vi "Process Data.vi"(8 "error in (no error)":errorcluster, 10 "Data In":string, 11 "Data Cluster in":T1={"Data Display"="", "FP Control Refs"={"Connect to Station Ref"=refnum, "Download Ref"=refnum, "Exit Button Ref"=refnum, "Start Date Refnum"=refnum, "End Date Refnum"=refnum, "Path"=refnum, "COM Port"="", "IP or Phone Ref"=refnum, "TCPIP ID"=refnum, "Reboot Refnum"=refnum, "Datafile Refnum"=refnum}, "FP Indicator Refs"={"Connected Refnum"=refnum, "Data Display Ref"=refnum, "Station ID Ref"=refnum}, "User Events"={"Stop"=refnum, "Update Display"=refnum}, "Message Queues"={"UI"=refnum, "ACQUISITION"=refnum, "PROCESSING"=refnum, "LOGGING"=refnum}, "IS IP?"=FALSE, "Downloading?"=FALSE, "DCP Version"=enum."XPert2", "Processing Loop State"=enum."Get Station  ID", "Username"=refnum, "Password"=refnum}) -> (0 "error out":errorcluster, 3 "Data Cluster out":T1={"Data Display"="", "FP Control Refs"={"Connect to Station Ref"=refnum, "Download Ref"=refnum, "Exit Button Ref"=refnum, "Start Date Refnum"=refnum, "End Date Refnum"=refnum, "Path"=refnum, "COM Port"="", "IP or Phone Ref"=refnum, "TCPIP ID"=refnum, "Reboot Refnum"=refnum, "Datafile Refnum"=refnum}, "FP Indicator Refs"={"Connected Refnum"=refnum, "Data Display Ref"=refnum, "Station ID Ref"=refnum}, "User Events"={"Stop"=refnum, "Update Display"=refnum}, "Message Queues"={"UI"=refnum, "ACQUISITION"=refnum, "PROCESSING"=refnum, "LOGGING"=refnum}, "IS IP?"=FALSE, "Downloading?"=FALSE, "DCP Version"=enum."XPert2", "Processing Loop State"=enum."Get Station  ID", "Username"=refnum, "Password"=refnum})   [LabVIEW 2018]
uses:
  controls/GLDL UI Data.ctl
  controls/Disconnect Control.ctl
  controls/Download Control.ctl
  controls/Exit Control.ctl
  controls/Date Control.ctl
  controls/IP Phone Number Control.ctl
  controls/Reboot Control.ctl
  controls/Connected Indicator.ctl
  controls/Output Indicator.ctl
  controls/Station ID Indicator.ctl
  Message Queue/All Message Queues.ctl
  Message Queue/Message Cluster.ctl
  controls/Processing Loop State.ctl
  Message Queue/Enqueue Message (Single).vi
  Message Queue/GLDL Message Queue.lvlib
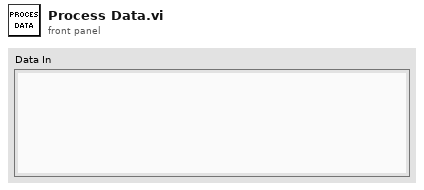
[diagram p1: front panel]
types:
  T1 = typedef "GLDL UI Data.ctl" = cluster{"Data Display":string, "FP Control Refs":cluster{"Connect to Station Ref":refnum<vi>, "Download Ref":refnum<vi>, "Exit Button Ref":refnum<vi>, "Start Date Refnum":refnum<vi>, "End Date Refnum":refnum<vi>, "Path":refnum<vi>, "COM Port":refnum<visa-resource-name>, "IP or Phone Ref":refnum<vi>, "TCPIP ID":refnum<k5>, "Reboot Refnum":refnum<vi>, "Datafile Refnum":refnum<file>}, "FP Indicator Refs":cluster{"Connected Refnum":refnum<vi>, "Data Display Ref":refnum<vi>, "Station ID Ref":refnum<vi>}, "User Events":cluster{"Stop":refnum<user-event>, "Update Display":refnum<user-event>}, "Message Queues":T2, "IS IP?":bool, "Downloading?":bool, "DCP Version":enum16{"XPert", "XPert2"}, "Processing Loop State":T3, "Username":refnum<vi>, "Password":refnum<vi>}
  T2 = typedef "GLDL Message Queue.lvlib/All Message Queues.ctl" = cluster{"UI":refnum<queue>, "ACQUISITION":refnum<queue>, "PROCESSING":refnum<queue>, "LOGGING":refnum<queue>}
  T3 = typedef "Processing Loop State.ctl" = enum16{"Get Station  ID", "Change Directory SD Card", "Change Directory Storage Card", "Downloading", "Idle in DL Directory"}
  T4 = typedef "Connected Indicator.ctl" = bool
  T5 = enum16{"open", "replace", "create", "open or create", "replace or create", "replace or create with confirmation"}
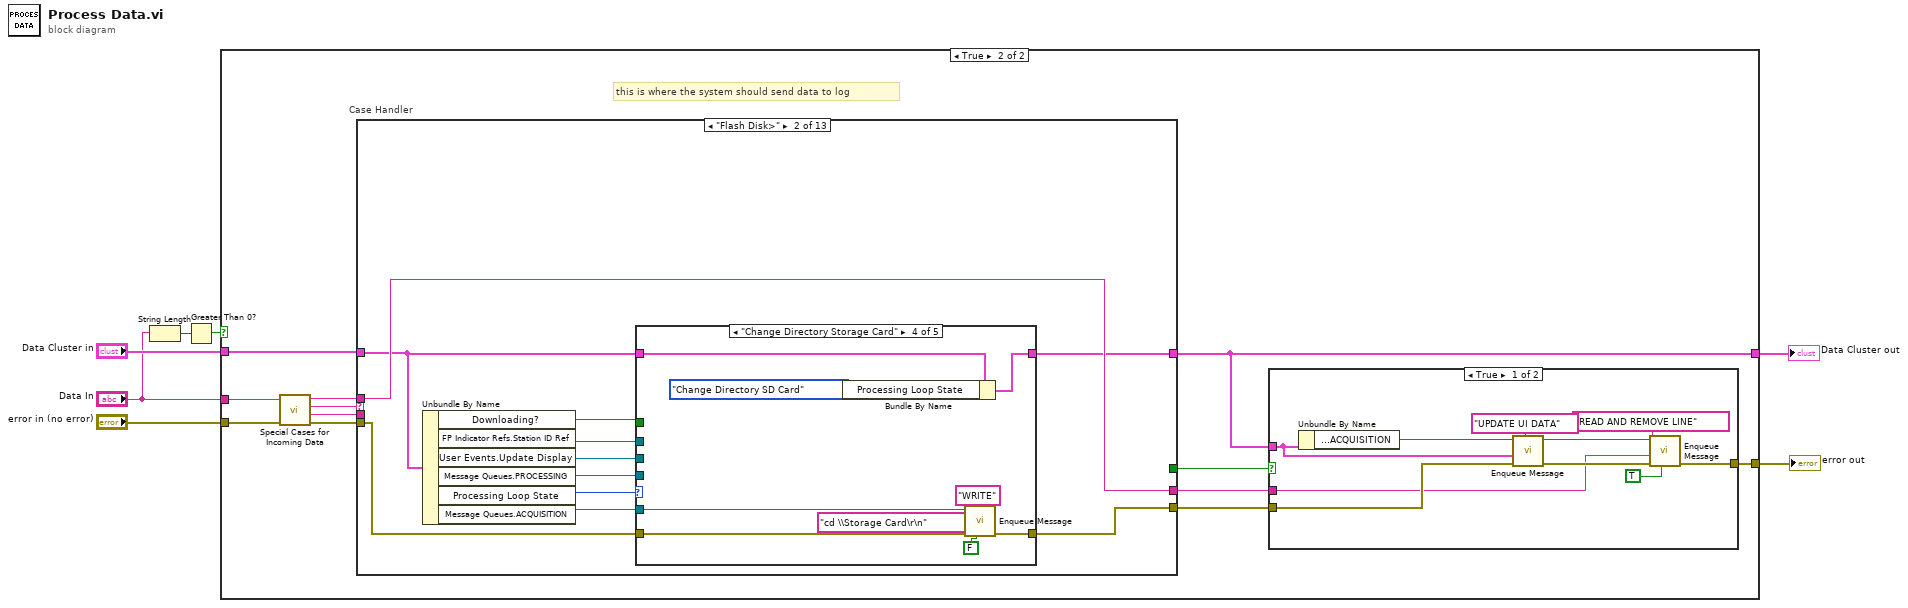
[diagram p0: block diagram]
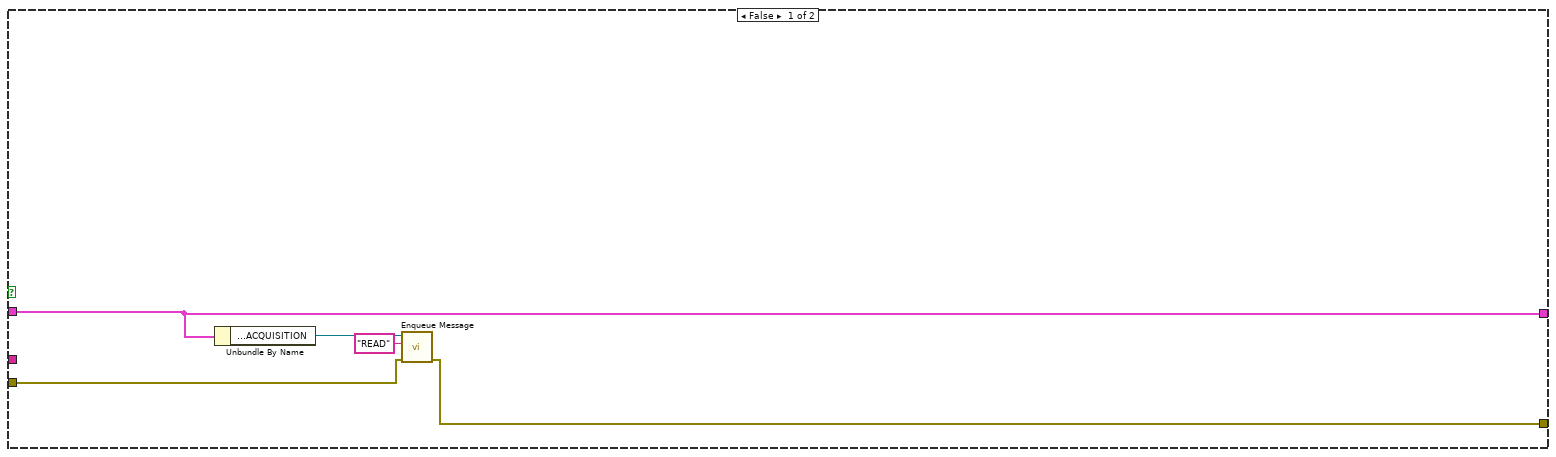
[diagram p2: hidden frame]
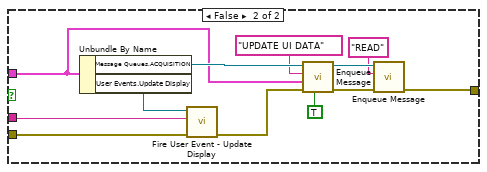
[diagram p3: hidden frame]
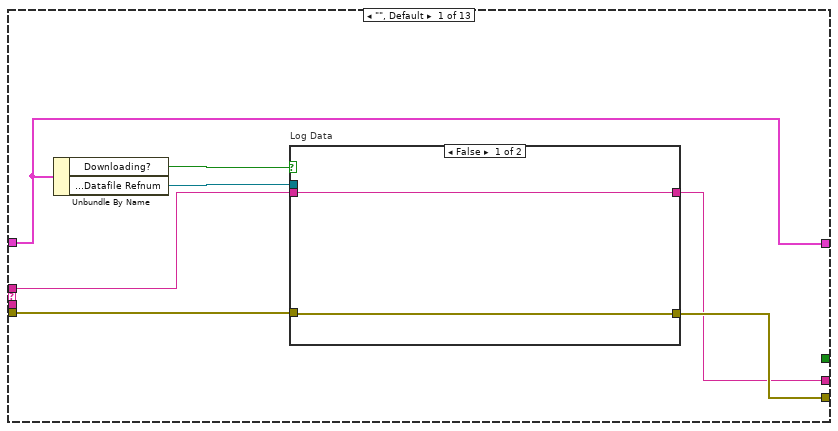
[diagram p4: hidden frame]
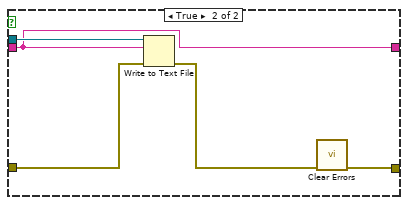
[diagram p5: hidden frame]
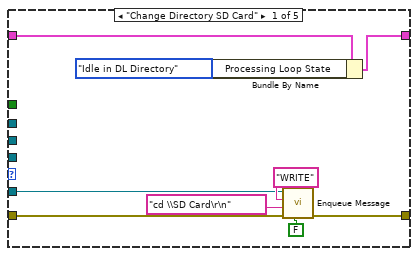
[diagram p6: hidden frame]
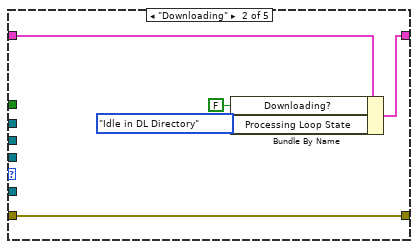
[diagram p7: hidden frame]
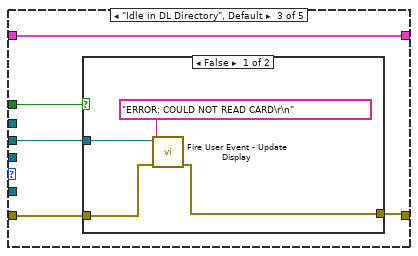
[diagram p8: hidden frame]
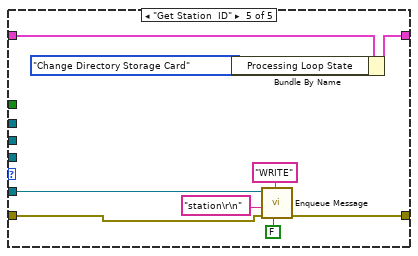
[diagram p10: hidden frame]
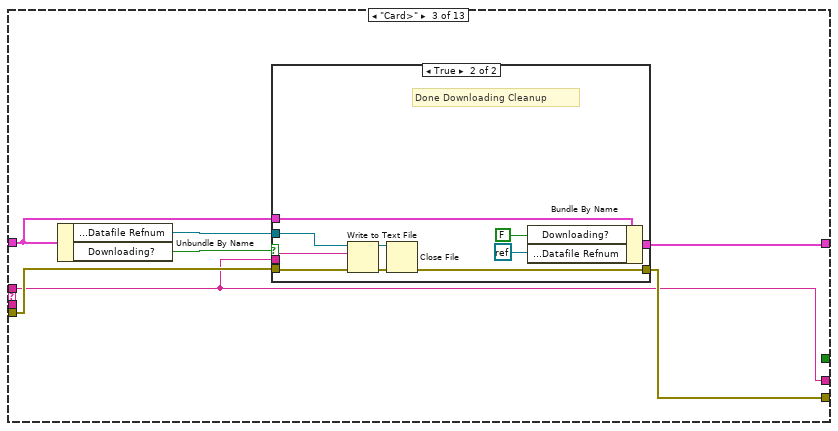
[diagram p11: hidden frame]
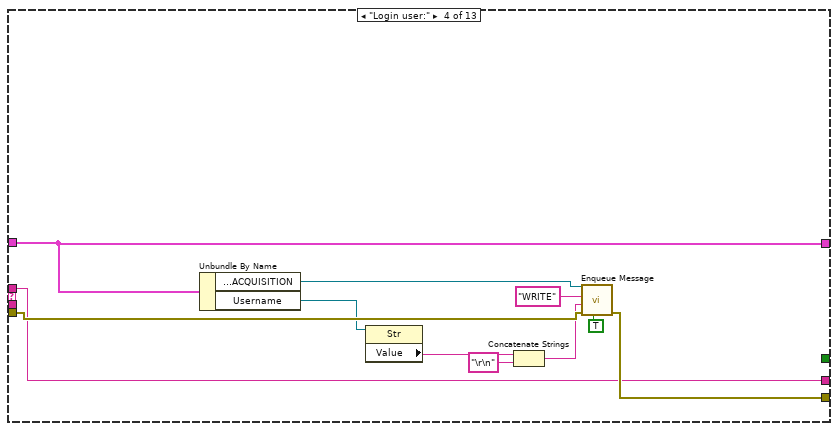
[diagram p13: hidden frame]
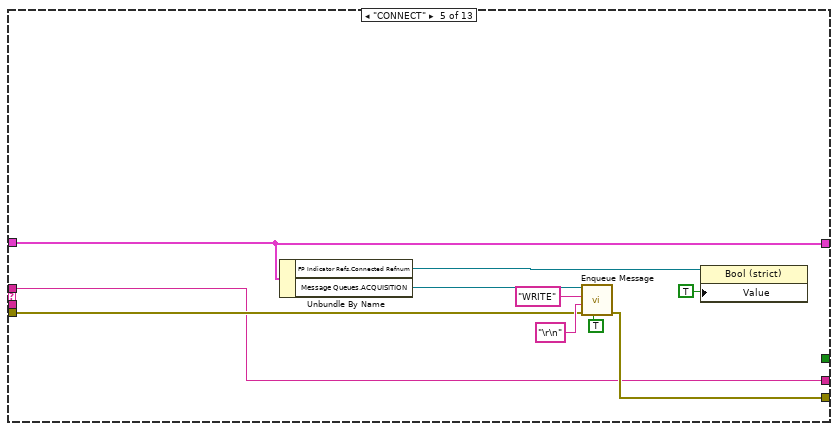
[diagram p14: hidden frame]
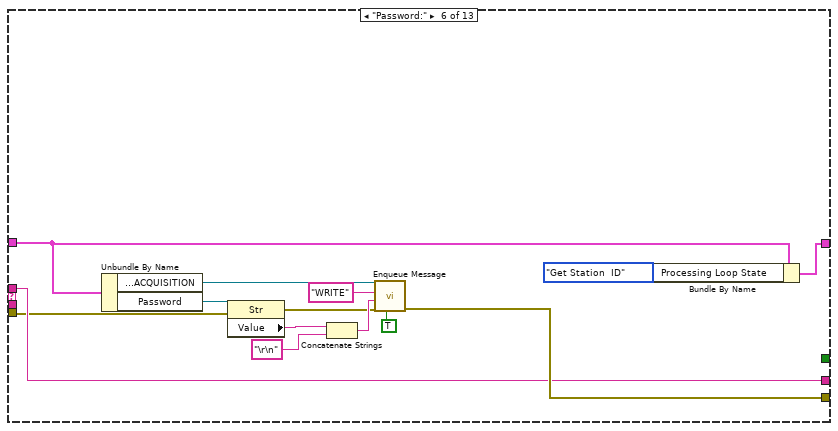
[diagram p15: hidden frame]
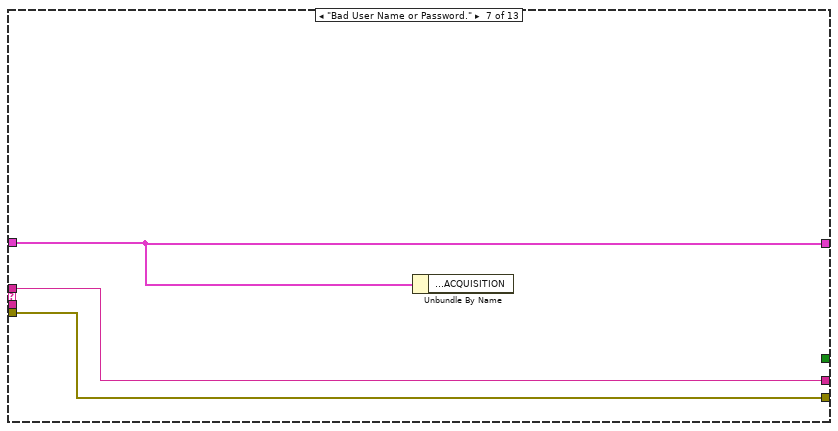
[diagram p16: hidden frame]
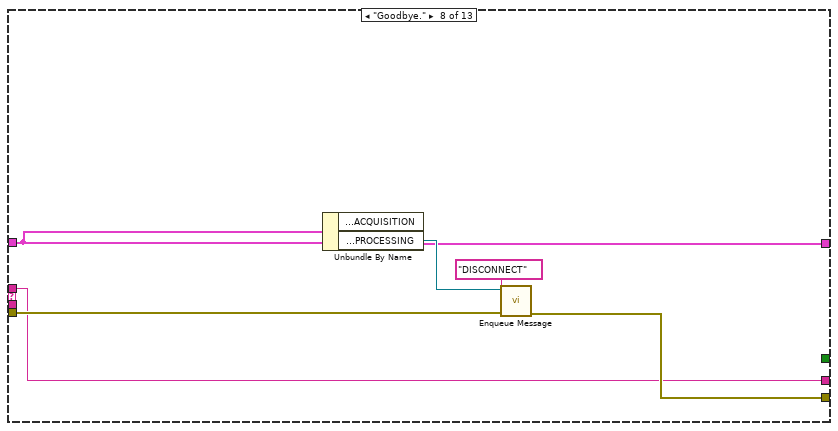
[diagram p17: hidden frame]
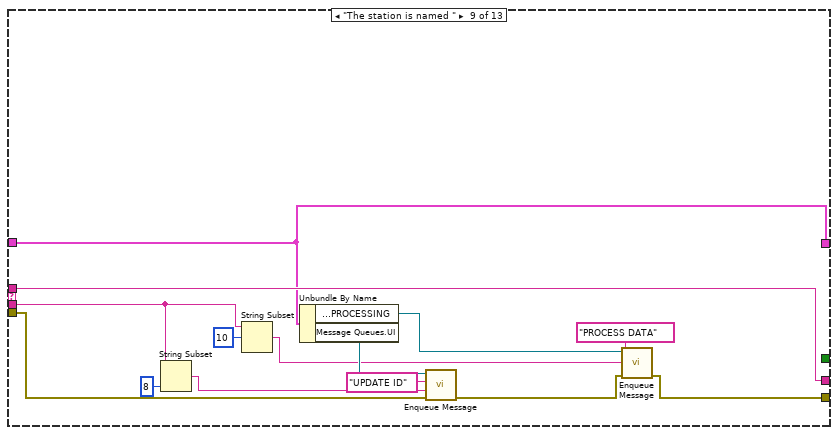
[diagram p18: hidden frame]
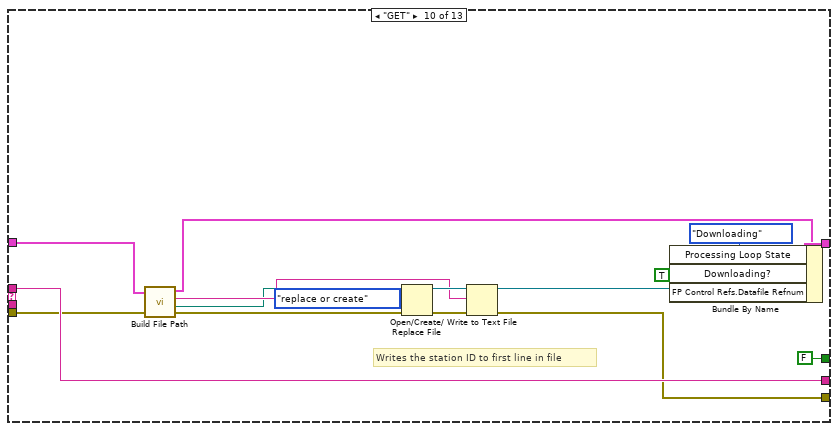
[diagram p19: hidden frame]
diagram:
  n1 = String Length(string="Data In") -> (length=w3:i32)
  n2 = Greater Than 0?(x=w3) -> (x > 0?=w2:bool)
  n3 = case shown="True" w2 {
    tunnel: "error in (no error)" -> [w9 w20]
    tunnel: [w8 w24] -> w5
    tunnel: "Data In" -> [_ w23]
    tunnel: "Data Cluster in" -> [w12 w18]
    tunnel: [w12 w13] -> w7
    frame False {
      n4 = Unbundle By Name(w12) -> ("Message Queues.ACQUISITION"=w11:refnum<queue>)
      n5 = call-poly "Enqueue Message.vi"("error in (no error)"=w9, "Message"="READ", "Message Queue"=w11) -> ("error out"=w8:errorcluster)  [unwired: 7 in, 1 out]
    }
    frame True {
      # "this is where the system should send data to log"
      n6 = call "Special Cases for Incoming Data.vi"("error in (no error)"=w20, "Data In"=w23) -> ("error out"=w22:errorcluster, "After Special Case"=w16:string, "Special Case"=w15:string, "Data Out"=w21:string)  [unwired: 5 in, 1 out]
      n7 = case "Case Handler" shown="\"Flash Disk>\"" w15 {
        tunnel: w22 -> [w50 w71 w116 w140 w149 w154 w170 w176 w185 w201 w207 w214 w225]
        tunnel: [w49 w63 w115 w141 w150 w165 w170 w174 w177 w193 w207 w213 w223] -> w17
        tunnel: w21 -> [w48 w69 w114 w137 w146 w163 w168 w171 w190 w206 w209 w219 w228]
        tunnel: w18 -> [w53 w66 w119 w139 w148 w162 w169 w172 w184 w203 w208 w218 w227]
        tunnel: [w47 w69 w114 w137 w146 w163 w168 w171 w190 w206 w209 w217 w228] -> w19
        tunnel: [w53 w65 w118 w139 w148 w161 w169 w172 w184 w204 w208 w218 w227] -> w13
        tunnel: w16 -> [_ _ _ _ _ _ _ _ w181 _ _ _ _]
        tunnel: [_ _ _ _ _ _ _ _ _ FALSE _ TRUE _] -> w14
        frame "", Default {
          n8 = Unbundle By Name(w53) -> ("Downloading?"=w52:bool, "FP Control Refs.Datafile Refnum"=w51:refnum<file>)
          n9 = case "Log Data" shown="False" w52 {
            tunnel: w51 -> [_ w60]
            tunnel: w50 -> [w55 w59]
            tunnel: [w55 w56] -> w49
            tunnel: w48 -> [w54 w58]
            tunnel: [w54 w58] -> w47
            frame False {
            }
            frame True {
              n10 = Write to Text File(file (use dialog)=w60, text=w58, error in=w59) -> (error out=w57:errorcluster)  [unwired: 1 in, 2 out]
              n11 = call <vilib>:"Clear Errors.vi"("error in (no error)"=w57) -> ("error out"=w56:errorcluster)  [unwired: 5 in, 1 out]
            }
          }
        }
        frame "Flash Disk>" {
          # "Get Station Number"
          n12 = Unbundle By Name(w66) -> ("Downloading?"=w61:bool, "FP Indicator Refs.Station ID Ref"=w62:refnum<vi>, "User Events.Update Display"=w64:refnum<user-event>, "Message Queues.PROCESSING"=w67:refnum<queue>, "Processing Loop State"=w68:T3, "Message Queues.ACQUISITION"=w70:refnum<queue>)
          n13 = case shown="\"Change Directory Storage Card\"" w68 {
            tunnel: w71 -> [w72 w85 w88 w96 w105]
            tunnel: w70 -> [w73 _ _ w97 w106]
            tunnel: [w74 w85 w87 w98 w107] -> w63
            tunnel: w67 -> [_ _ _ _ _]
            tunnel: w66 -> [w80 w84 w90 w104 w112]
            tunnel: [w79 w83 w90 w103 w113] -> w65
            tunnel: w64 -> [_ _ w89 _ _]
            tunnel: w62 -> [_ _ _ _ _]
            tunnel: w61 -> [_ _ w86 _ _]
            frame "Change Directory SD Card" {
              n14 = Bundle By Name(cluster=w80, "Processing Loop State"=Processing_Loop_State."Idle in DL Directory") -> (w79:T1)
              n15 = call-poly "Enqueue Message.vi"("Priority Message? (F)"=FALSE, "error in (no error)"=w72, "Message Data"="cd \\SD Card\r\n" ("Initial Message"), "Message"="WRITE" ("Initial Message"), "Message Queue"=w73) -> ("error out"=w74:errorcluster)  [unwired: 5 in, 1 out]
            }
            frame "Downloading" {
              n16 = Bundle By Name(cluster=w84, "Downloading?"=FALSE, "Processing Loop State"=Processing_Loop_State."Idle in DL Directory") -> (w83:T1)
            }
            frame "Idle in DL Directory", Default {
              n17 = case shown="False" w86 {
                tunnel: w89 -> [w94 _]
                tunnel: w88 -> [w93 w95]
                tunnel: [w91 w95] -> w87
                frame False {
                  n18 = call "Fire User Event - Update Display.vi"("error in (no error)"=w93, "event data"="ERROR: COULD NOT READ CARD\r\n" ("Initial Message"), "Update Display"=w94) -> ("error out"=w91:errorcluster)  [unwired: 8 in]
                }
                frame True {
                }
              }
            }
            frame "Change Directory Storage Card" {
              n19 = Bundle By Name(cluster=w104, "Processing Loop State"=Processing_Loop_State."Change Directory SD Card") -> (w103:T1)
              n20 = call-poly "Enqueue Message.vi"("Priority Message? (F)"=FALSE, "error in (no error)"=w96, "Message Data"="cd \\Storage Card\r\n" ("data in"), "Message"="WRITE" ("Initial Message"), "Message Queue"=w97) -> ("error out"=w98:errorcluster)  [unwired: 5 in, 1 out]
            }
            frame "Get Station  ID" {
              n21 = Bundle By Name(cluster=w112, "Processing Loop State"=Processing_Loop_State."Change Directory Storage Card") -> (w113:T1)
              n22 = call-poly "Enqueue Message.vi"("Priority Message? (F)"=FALSE, "error in (no error)"=w105, "Message Data"="station\r\n" ("data in"), "Message"="WRITE" ("Initial Message"), "Message Queue"=w106) -> ("error out"=w107:errorcluster)  [unwired: 5 in, 1 out]
            }
          }
        }
        frame "Card>" {
          n23 = Unbundle By Name(w119) -> ("FP Control Refs.Datafile Refnum"=w117:refnum<file>, "Downloading?"=w120:bool)
          n24 = case shown="True" w120 {
            tunnel: w119 -> [w122 w132]
            tunnel: [w122 w130] -> w118
            tunnel: w117 -> [_ w128]
            tunnel: w116 -> [w121 w125]
            tunnel: [w121 w124] -> w115
            tunnel: w114 -> [_ w123]
            frame False {
              # "Not Done Downloading"
            }
            frame True {
              # "Done Downloading Cleanup"
              n25 = Write to Text File(file (use dialog)=w128, text=w123, error in=w125) -> (refnum out=w127:refnum<file>, error out=w126:errorcluster)  [unwired: 1 in, 1 out]
              n26 = Close File(refnum=w127, error in=w126) -> (error out=w124:errorcluster)  [unwired: 1 out]
              n27 = Bundle By Name(cluster=w132, "Downloading?"=FALSE, "FP Control Refs.Datafile Refnum"=refnum<k0> refnum) -> (w130:T1)
            }
          }
        }
        frame "Login user:" {
          n28 = Unbundle By Name(w139) -> ("Message Queues.ACQUISITION"=w138:refnum<queue>, "Username"=w136:refnum<vi>)
          n29 = property class="Str"(reference=w136) -> ("Value"=w135:string)  [unwired: 1 in, 2 out]
          n30 = Concatenate Strings(w135, "\r\n" ("write buffer")) -> (w133:string)
          n31 = call-poly "Enqueue Message.vi"("Priority Message? (F)"=TRUE, "error in (no error)"=w140, "Message Data"=w133, "Message"="WRITE" ("Initial Message"), "Message Queue"=w138) -> ("error out"=w141:errorcluster)  [unwired: 5 in, 1 out]
        }
        frame "CONNECT" {
          n32 = Unbundle By Name(w148) -> ("FP Indicator Refs.Connected Refnum"=w145:refnum<vi>, "Message Queues.ACQUISITION"=w147:refnum<queue>)
          n33 = call-poly "Enqueue Message.vi"("Priority Message? (F)"=TRUE, "error in (no error)"=w149, "Message Data"="\r\n" ("write buffer"), "Message"="WRITE" ("Initial Message"), "Message Queue"=w147) -> ("error out"=w150:errorcluster)  [unwired: 5 in, 1 out]
          n34 = property class="Bool (strict)"(reference=w145, "Value"=T4 TRUE) -> ()  [unwired: 1 in, 2 out]
        }
        frame "Password:" {
          # "akl is the only option for now"
          n35 = Unbundle By Name(w162) -> ("Message Queues.ACQUISITION"=w164:refnum<queue>, "Password"=w159:refnum<vi>)
          n36 = property class="Str"(reference=w159, error in=w154) -> (error out=w155:errorcluster, "Value"=w158:string)  [unwired: 1 out]
          n37 = Concatenate Strings(w158, "\r\n" ("write buffer")) -> (w156:string)
          n38 = call-poly "Enqueue Message.vi"("Priority Message? (F)"=TRUE, "error in (no error)"=w155, "Message Data"=w156, "Message"="WRITE" ("Initial Message"), "Message Queue"=w164) -> ("error out"=w165:errorcluster)  [unwired: 5 in, 1 out]
          n39 = Bundle By Name(cluster=w162, "Processing Loop State"=Processing_Loop_State."Get Station  ID") -> (w161:T1)
        }
        frame "Bad User Name or Password." {
          n40 = Unbundle By Name(w169) -> ()  [unwired: 1 out]
        }
        frame "Goodbye." {
          # "Logged out. Now Disconnect"
          n41 = Unbundle By Name(w172) -> ("Message Queues.PROCESSING"=w173:refnum<queue>)  [unwired: 1 out]
          n42 = call-poly "Enqueue Message.vi"("error in (no error)"=w176, "Message"="DISCONNECT", "Message Queue"=w173) -> ("error out"=w174:errorcluster)  [unwired: 7 in, 1 out]
        }
        frame "The station is named " {
          # "Do something with the Station ID"
          n43 = String Subset(string=w181, length (rest)=8 ("length (rest)")) -> (substring=w188:string)  [unwired: 1 in]
          n44 = String Subset(string=w181, offset (0)=10) -> (substring=w179:string)  [unwired: 1 in]
          n45 = Unbundle By Name(w184) -> ("Message Queues.PROCESSING"=w182:refnum<queue>, "Message Queues.UI"=w187:refnum<queue>)
          n46 = call-poly "Enqueue Message.vi"("error in (no error)"=w185, "Message Data"=w188, "Message"="UPDATE ID", "Message Queue"=w187) -> ("error out"=w178:errorcluster)  [unwired: 6 in, 1 out]
          n47 = call-poly "Enqueue Message.vi"("error in (no error)"=w178, "Message Data"=w179, "Message"="PROCESS DATA", "Message Queue"=w182) -> ("error out"=w177:errorcluster)  [unwired: 6 in, 1 out]
        }
        frame "GET" {
          # "Writes the station ID to first line in file"
          n48 = call "Build File Path.vi"("error in (no error)"=w201, "Data Cluster in"=w203) -> ("error out"=w202:errorcluster, "appended path"=w196:path, "Station ID"=w197:string, "Data Cluster out"=w194:T1)  [unwired: 6 in]
          n49 = Open/Create/Replace File(file path (use dialog)=w196, error in=w202, operation (0:open)=T5."replace or create") -> (refnum out=w200:refnum<file>, error out=w199:errorcluster)  [unwired: 3 in, 1 out]
          n50 = Write to Text File(file (use dialog)=w200, text=w197, error in=w199) -> (refnum out=w198:refnum<file>, error out=w193:errorcluster)  [unwired: 1 in, 1 out]
          n51 = Bundle By Name(cluster=w194, "Processing Loop State"=Processing_Loop_State."Downloading", "Downloading?"=TRUE, "FP Control Refs.Datafile Refnum"=w198) -> (w204:T1)
        }
        frame ".LOG" {
        }
        frame "-- More --" {
          # "Spacebar ASCII Code(U8)"
          # "Remove the -- More -- \nfrom the string."
          # "Tell Acquisition loop to Get More Data"
          n52 = String Length(string=w219) -> (length=w222:i32)
          n53 = Subtract(x=w222, y=11 ("length (rest)")) -> (x-y=w221:i32)
          n54 = String Subset(string=w219, length (rest)=w221) -> (substring=w217:string)  [unwired: 1 in]
          n55 = Unbundle By Name(w218) -> ("Message Queues.ACQUISITION"=w215:refnum<queue>)
          n56 = Type Cast(x=u8 32 ("timeout ms (25000)")) -> (*(type *) &x=w211:string)  [unwired: 1 in]
          n57 = call-poly "Enqueue Message.vi"("error in (no error)"=w214, "Message Data"=w211, "Message"="WRITE" ("Initial Message"), "Message Queue"=w215) -> ("error out"=w213:errorcluster)  [unwired: 6 in, 1 out]
        }
        frame "NO CARRIER" {
          n58 = Unbundle By Name(w227) -> ("Message Queues.ACQUISITION"=w226:refnum<queue>)
          n59 = call-poly "Enqueue Message.vi"("error in (no error)"=w225, "Message"="DISCONNECT" ("Initial Message"), "Message Queue"=w226) -> ("error out"=w223:errorcluster)  [unwired: 7 in, 1 out]
        }
      }
      n60 = case shown="True" w14 {
        tunnel: [w33 w38] -> w24
        tunnel: w19 -> [w25 w46]
        tunnel: w17 -> [w31 w45]
        tunnel: w13 -> [w29 w40]
        frame True {
          n61 = Unbundle By Name(w29) -> ("Message Queues.ACQUISITION"=w30:refnum<queue>)
          n62 = call-poly "Enqueue Message.vi"("error in (no error)"=w31, "Message Data"=w29, "Message"="UPDATE UI DATA" ("Initial Message"), "Message Queue"=w30) -> ("error out"=w32:errorcluster, "dup Message Queue"=w27:refnum<queue>)  [unwired: 6 in]
          n63 = call-poly "Enqueue Message.vi"("Priority Message? (F)"=TRUE, "error in (no error)"=w32, "Message Data"=w25, "Message"="READ AND REMOVE LINE" ("Initial Message"), "Message Queue"=w27) -> ("error out"=w33:errorcluster)  [unwired: 5 in, 1 out]
        }
        frame False {
          n64 = Unbundle By Name(w40) -> ("Message Queues.ACQUISITION"=w43:refnum<queue>, "User Events.Update Display"=w44:refnum<user-event>)
          n65 = call "Fire User Event - Update Display.vi"("error in (no error)"=w45, "event data"=w46, "Update Display"=w44) -> ("error out"=w41:errorcluster)  [unwired: 8 in]
          n66 = call-poly "Enqueue Message.vi"("Priority Message? (F)"=TRUE, "error in (no error)"=w41, "Message Data"=w40, "Message"="UPDATE UI DATA" ("Initial Message"), "Message Queue"=w43) -> ("error out"=w39:errorcluster, "dup Message Queue"=w37:refnum<queue>)  [unwired: 5 in]
          n67 = call-poly "Enqueue Message.vi"("error in (no error)"=w39, "Message"="READ" ("Initial Message"), "Message Queue"=w37) -> ("error out"=w38:errorcluster)  [unwired: 7 in, 1 out]
        }
      }
    }
  }
  "Data Cluster out" <- w7
  "error out" <- w5
